vi "Configure IP Address.vi"(0 "VISA resource name":refnum<visa-resource-name>, 5 "IP Address":string="100.100.100.100", 11 "error in (no error)":errorcluster) -> (4 "VISA resource name out":refnum<visa-resource-name>, 15 "error out":errorcluster)   [LabVIEW 2012, in "Associated Research 78XX Series.lvlib"]
doc: "Sets the IP Address Of the APT 6000 Series Power Source instrument\n\nNote: This setting is supported for <B>Firmware Version 2.0</B> Only"
uses:
  <instrlib>/Associated Research 78XX Series/Associated Research 78XX Series.lvlib
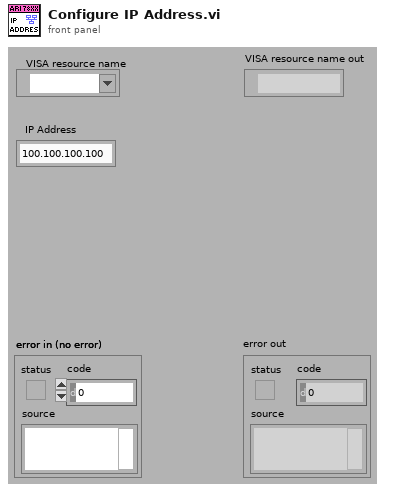
[diagram p1: front panel]
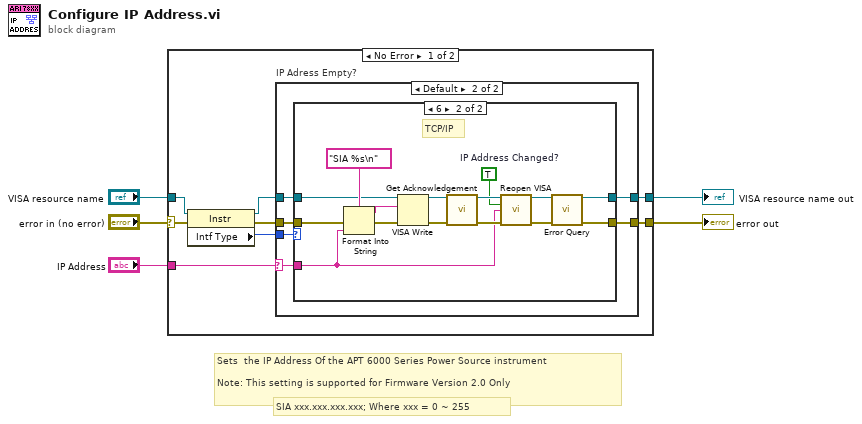
[diagram p0: block diagram]
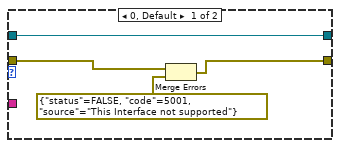
[diagram p3: hidden frame]
diagram:
  # "SIA xxx.xxx.xxx.xxx; Where xxx = 0 ~ 255"
  # "Sets  the IP Address Of the APT 6000 Series Power Source instrument\n\nNote: This setting is supported for Firmware Version 2.0 Only"
  n1 = case shown="No Error" "error in (no error)" {
    selector: "error in (no error)" -> [w11 w42]
    tunnel: "VISA resource name" -> [w9 w41]
    tunnel: [w13 w41] -> w5
    tunnel: [w12 w42] -> w4
    tunnel: "IP Address" -> [w6 _]
    frame No Error {
      n2 = property class="Instr"(reference=w9, error in=w11) -> (reference out=w8:refnum<visa-resource-name>, error out=w10:errorcluster, "Intf Type"=w7:u16)
      n3 = case "IP Adress Empty?" shown="Default" w6 {
        selector: w6 -> [_ w16]
        tunnel: [w14 w21] -> w13
        tunnel: [w15 w20] -> w12
        tunnel: w10 -> [w15 w19]
        tunnel: w8 -> [w14 w18]
        tunnel: w7 -> [_ w17]
        frame "" {
        }
        frame Default {
          n4 = case shown="6" w17 {
            tunnel: [w25 w40] -> w21
            tunnel: [w23 w38] -> w20
            tunnel: w19 -> [w22 w32]
            tunnel: w18 -> [w25 w31]
            tunnel: w16 -> [_ w26]
            frame 0, Default {
              n5 = Merge Errors(w22, errorcluster {"status"=FALSE, "code"=5001, "source"="This Interface not supported"} ("error in 2 (no error)")) -> (w23:errorcluster)
            }
            frame 6 {
              w27 = TRUE  # IP Address Changed?
              # "TCP/IP"
              n6 = Format Into String(format string="SIA %s\n" ("Command to Send"), error in=w32, w26) -> (resulting string=w37:string, error out=w36:errorcluster)  [unwired: 1 in]
              n7 = VISA Write(VISA resource name=w31, write buffer=w37, error in (no error)=w36) -> (VISA resource name out=w33:refnum<visa-resource-name>, error out=w39:errorcluster)  [unwired: 1 out]
              n8 = call <instrlib>:"Get Acknowledgement.vi"("VISA resource name"=w33, "error in (no error)"=w39) -> ("VISA resource name out"=w29:refnum<visa-resource-name>, "error out"=w34:errorcluster)  [unwired: 12 in]
              n9 = call <instrlib>:"Reopen VISA.vi"("VISA resource name"=w29, "IP Address Changed (F)?"=w27, "IP Address (000.000.000.000)"=w26, "error in (no error)"=w34) -> ("VISA resource name out"=w28:refnum<visa-resource-name>, "error out"=w30:errorcluster)  [unwired: 10 in]
              n10 = call <instrlib>:"Error Query.vi"("VISA resource name"=w28, "error in (no error)"=w30) -> ("VISA resource name out"=w40:refnum<visa-resource-name>, "error out"=w38:errorcluster)  [unwired: 10 in, 2 out]
            }
          }
        }
      }
    }
    frame Error {
    }
  }
  "error out" <- w4
  "VISA resource name out" <- w5
